vi "Hold.vi"(8 "error in (no error)":errorcluster, 9 "hold (0:off)":u32(ring) items=["off", "on", "trigger"], 11 "VISA resource name":refnum<visa-resource-name>) -> (0 "error out":errorcluster, 3 "VISA resource name out":refnum<visa-resource-name>)   [LabVIEW 2020, in "Agilent 6XXX Series.lvlib"]
doc: "This function controls the hold feature of the instrument. Using this function, commands may be held for future implemention and previously held commands may be triggered. This function is valid for the HP603XA series only."
uses:
  <instrlib>/Agilent 6XXX Series/Agilent 6XXX Series.lvlib
panel:
  # "HP603XA series only"
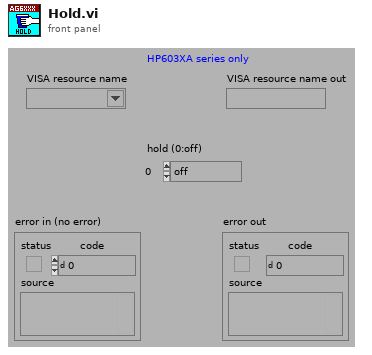
[diagram p1: front panel]
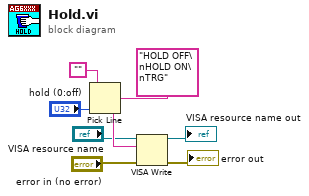
[diagram p0: block diagram]
diagram:
  n1 = Pick Line(string ("")="", multi-line string="HOLD OFF\nHOLD ON\nTRG", line index="hold (0:off)") -> (output string=w5:string)
  n2 = VISA Write(VISA resource name="VISA resource name", write buffer=w5, error in (no error)="error in (no error)") -> (VISA resource name out=→"VISA resource name out":refnum<visa-resource-name>, error out=→"error out":errorcluster)  [unwired: 1 out]
